vi "Test Controller To Not Terminate if Not Verified.vi"(8 "error in (no error)":errorcluster, 11 "Test Case In":refnum<class "Controller Test.lvclass">) -> (0 "error out":errorcluster, 3 "Test Case Out":refnum<class "Controller Test.lvclass">)   [LabVIEW 2020, in "Controller Test.lvclass"]
uses:
  Controller Test.lvclass
  C:/Program Files (x86)/National Instruments/LabVIEW 2020/vi.lib/Astemes/LUnit/Test Case.lvclass
  ATM Controller/State.ctl
  <vilib>/Astemes/LUnit/Test Case.lvclass/Test Case.ctl
  01074fa8-ee8a-411d-bc8b-fc92c4f90959.vi
  <vilib>/Astemes/LUnit/Palette/Pass.vi
  <vilib>/Astemes/LUnit/Palette/Fail.vi
  <vilib>/Astemes/LUnit/Compare Variants.vi
  <vilib>/Astemes/LUnit/Describe Comparison.vi
  <vilib>/Astemes/LUnit/Set Assertion Type.vi
  <vilib>/Astemes/LUnit/Add test result.vi
  <vilib>/Astemes/LUnit/Variant to string.vi
  <vilib>/Astemes/LUnit/LUnit Record Assertion Result.vi
  <vilib>/Astemes/LUnit/LUnit Aggregate Assertion Results.vi
  <vilib>/Astemes/LUnit/Method Result/LUnit Merge Status.vi
  <vilib>/Astemes/LUnit/LUnit Concatenate result strings.vi
  <vilib>/Utility/Data Type/Get Type Information.vi
  <vilib>/Utility/LVClass/Get LV Class Name.vi
  Controller Test.lvclass/Controller Test.ctl
  ATM Controller/ATM Controller.lvclass
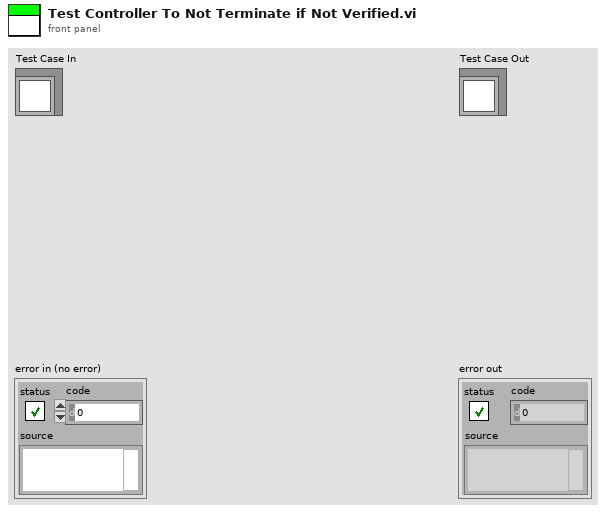
[diagram p1: front panel]
types:
  T1 = typedef "ATM Controller.lvclass/State.ctl" = enum16{"Start", "Card Inserted", "Verification Failed", "Verification Succeeded", "Depositing", "Depositing Completed", "Withdrawing", "Withdraw Completed", "Withdraw Failed", "Balance Inquiry", "Terminate"}
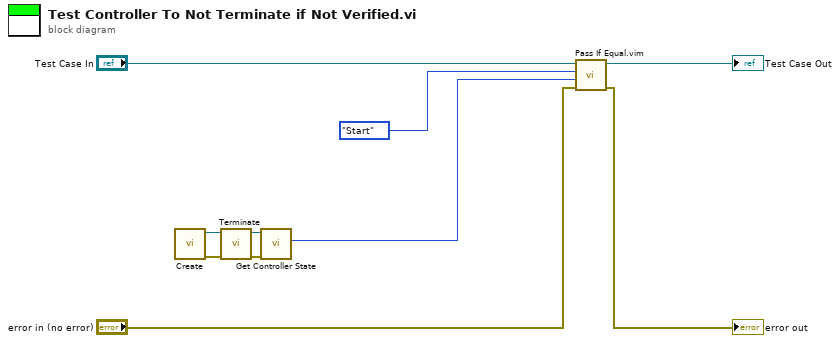
[diagram p0: block diagram]
diagram:
  n1 = call "Create.vi"() -> ("error out"=w1:errorcluster, "ATM Controller out"=w2:refnum<class "ATM Controller.lvclass">)  [unwired: 10 in]
  n2 = call "Terminate.vi"("error in (no error)"=w1, "ATM Controller in"=w2) -> ("error out"=w4:errorcluster, "ATM Controller out"=w3:refnum<class "ATM Controller.lvclass">)  [unwired: 8 in]
  n3 = call "Get Controller State.vi"("error in (no error)"=w4, "ATM Controller in"=w3) -> ("ATM State"=w6:T1)  [unwired: 7 in, 2 out]
  n4 = call "Pass If Equal.vim"("error in (no error)"="error in (no error)", "Actual"=w6, "Expected"=State."Start" ("ATM State"), "LUnit Test Case In"="Test Case In") -> ("error out"=→"error out":errorcluster, "LUnit Test Case Out"=→"Test Case Out":refnum<class "Controller Test.lvclass">)  [unwired: 6 in]
